vi "_CenterSizeToBoundingBox.vi"(10 "Size":T1, 11 "Center-Point":T1) -> (3 "Bounding Box":T2)   [LabVIEW 2020, in "OpenLvVision_Overlays.lvlib"]
doc: "Creates form a center and size a bounding box."
uses:
  OpenLvVision_Overlays.lvlib
  <vilib>/OpenLvVision/OpenLvVision_Image/DataAccess/TypeDef/OLV RectangleI32.ctl
  <vilib>/OpenLvVision/OpenLvVision_Image/DataAccess/OLV DataAccess.lvlib
  TypeDefs/PointI32.ctl
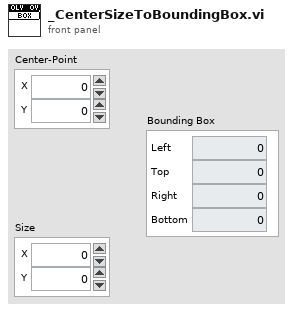
[diagram p1: front panel]
types:
  T1 = typedef "OpenLvVision_Overlays.lvlib/PointI32.ctl" = cluster{"X":i32, "Y":i32}
  T2 = typedef "OLV OpenLvVision_Image.lvlib/OLV DataAccess.lvlib/OLV RectangleI32.ctl" = cluster{"Left":i32, "Top":i32, "Right":i32, "Bottom":i32}
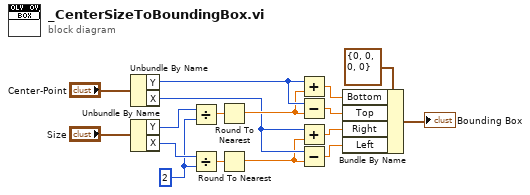
[diagram p0: block diagram]
diagram:
  w2 = 2
  n1 = Unbundle By Name("Center-Point") -> ("Y"=w12:i32, "X"=w10:i32)
  n2 = Unbundle By Name("Size") -> ("Y"=w16:i32, "X"=w17:i32)
  n3 = Divide(x=w16, y=w2) -> (x/y=w15:dbl)
  n4 = Divide(x=w17, y=w2) -> (x/y=w14:dbl)
  n5 = Round To Nearest(number=w15) -> (nearest integer value=w11:dbl)
  n6 = Round To Nearest(number=w14) -> (nearest integer value=w5:dbl)
  n7 = Add(x=w12, y=w11) -> (x+y=w9:dbl)
  n8 = Subtract(x=w12, y=w11) -> (x-y=w6:dbl)
  n9 = Add(x=w10, y=w5) -> (x+y=w7:dbl)
  n10 = Subtract(x=w10, y=w5) -> (x-y=w8:dbl)
  n11 = Bundle By Name(cluster=T2 {"Left"=0, "Top"=0, "Right"=0, "Bottom"=0} ("Rectangle"), "Bottom"=w9, "Top"=w6, "Right"=w7, "Left"=w8) -> (→"Bounding Box":T2)
